vi "ROI_array_to_cluster.vi"(11 "Camera Acquire Settings":T2) -> (3 "output cluster":T1)   [LabVIEW 2013]
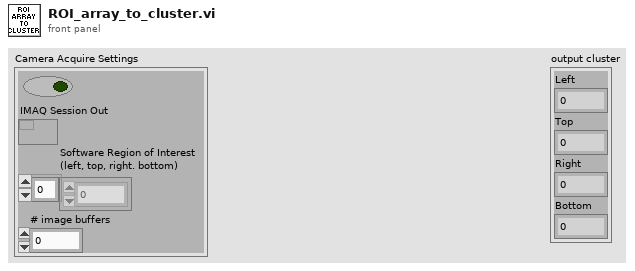
[diagram p1: front panel]
types:
  T1 = cluster{"Left":i32, "Top":i32, "Right":i32, "Bottom":i32}
  T2 = cluster{bool, "IMAQ Session Out":refnum<k11>, "Software Region of Interest\n(left, top, right. bottom)":i32[], "# image buffers":i32}
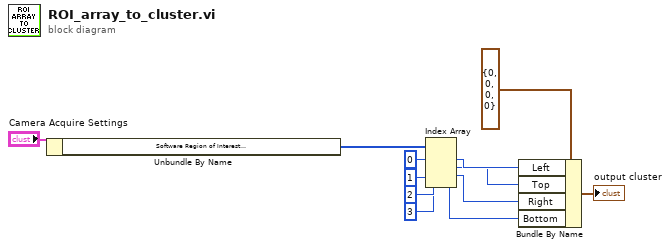
[diagram p0: block diagram]
diagram:
  n1 = Unbundle By Name("Camera Acquire Settings") -> ("Software Region of Interest\n(left, top, right. bottom)"=w11:i32[])
  n2 = Index Array(array=w11, index #1=0 ("index"), index #2=1 ("index"), index #3=2 ("index"), index #4=3 ("index")) -> (element #1=w5:i32, element #2=w4:i32, element #3=w3:i32, element #4=w2:i32)
  n3 = Bundle By Name(cluster=T1 {"Left"=0, "Top"=0, "Right"=0, "Bottom"=0} ("Rectangle"), "Left"=w5, "Top"=w4, "Right"=w3, "Bottom"=w2) -> (→"output cluster":T1)
